vi "asset.links.from_json.vi"(8 "error in":errorcluster, 10 "json":string) -> (0 "error out":errorcluster, 2 "Links":T1)   [LabVIEW 2020, in "Nominal Client.lvclass"]
uses:
  Nominal Client.lvclass
  links.ctl
  da3c3072-a0b3-4c36-a5a9-8b605c2a1e9f.vi
  <vilib>/JDP Science/JSONtext/JSON text to Variant.vi
  <vilib>/JDP Science/JSONtext/LVClass Serializer/JSONtext LVClass Serializer.lvclass
  Nominal Client.lvclass/Nominal Client.ctl
  nominal types/dataScope/dataScopes.lvlib
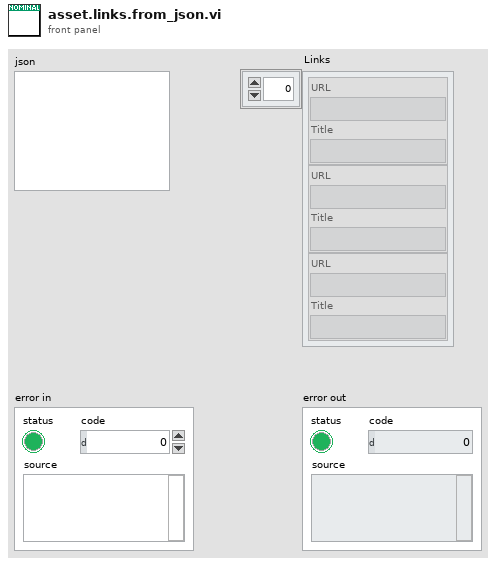
[diagram p1: front panel]
types:
  T1 = typedef "dataScopes.lvlib/links.ctl" = cluster{"URL":string, "Title":string}[]
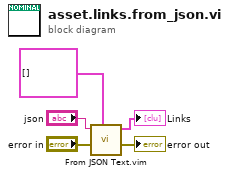
[diagram p0: block diagram]
diagram:
  n1 = call "From JSON Text.vim"("Data Type and Default Value"=cluster{"url":string, "title":string}[] [], "error in (no error)"="error in", "JSON"="json") -> ("error out"=→"error out":errorcluster, "Data out"=→"Links":cluster{"url":string, "title":string}[])  [unwired: 7 in]
